vi "FindFaces.vi"() -> ()   [LabVIEW 2018]
panel:
  out "Image to process":picture
  out "Processed image":picture
  out "Error":errorcluster
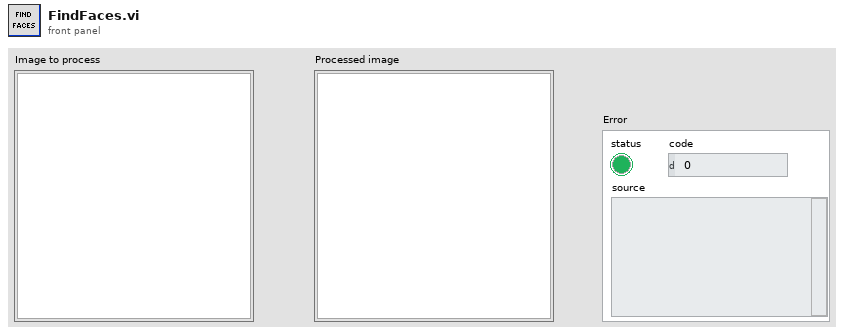
[diagram p1: front panel]
types:
  T1 = typedef "imagedata.ctl" = cluster{"image type":i32, "image depth":i32, "image":u8[], "mask":u8[], "colors":u32[], "Rectangle":cluster{"left":i16, "top":i16, "right":i16, "bottom":i16}}
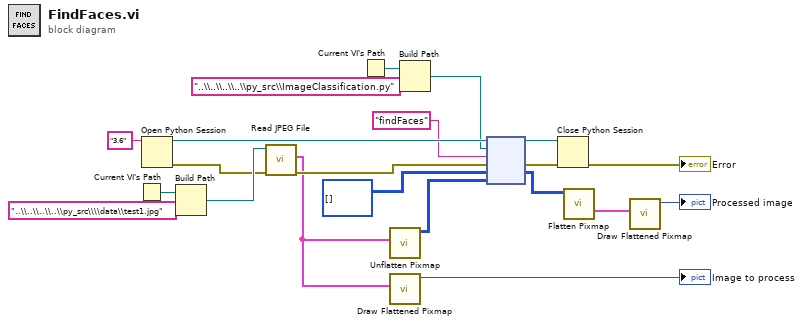
[diagram p0: block diagram]
diagram:
  n1 = Current VI's Path() -> (path=w12:path)
  n2 = Open Python Session(python version="3.6" ("Python version")) -> (session out=w21:refnum<k35>, error out=w7:errorcluster)  [unwired: 2 in]
  n3 = Build Path(base path=w12, name or relative path="..\\..\\..\\..\\py_src\\\\data\\test1.jpg") -> (appended path=w10:path)
  n4 = call <vilib>:"Read JPEG File.vi"("error in (no error)"=w7, "path to JPEG file"=w10) -> ("error out"=w6:errorcluster, "image data"=w4:T1)  [unwired: 7 in, 1 out]
  n5 = Current VI's Path() -> (path=w15:path)
  n6 = call <vilib>:"Unflatten Pixmap.vi"("image data"=w4) -> ("24-bit pixmap"=w1:u32[][])  [unwired: 4 in, 6 out]
  n7 = call <vilib>:"Draw Flattened Pixmap.vi"("image data"=w4) -> ("new picture"=→"Image to process":picture)  [unwired: 8 in]
  n8 = Build Path(base path=w15, name or relative path="..\\..\\..\\..\\py_src\\ImageClassification.py") -> (appended path=w13:path)
  n9 = node(w21, w13, "findFaces" ("function name"), w6, u32[][] [], w1) -> (w20:refnum<k35>, w19:errorcluster, w2:u32[][])  [unwired: 1 in, 2 out]
  n10 = Close Python Session(session in=w20, error in=w19) -> (11:→"Error":errorcluster)
  n11 = call <vilib>:"Flatten Pixmap.vi"("24-bit pixmap"=w2) -> ("image data"=w9:T1)  [unwired: 10 in]
  n12 = call <vilib>:"Draw Flattened Pixmap.vi"("image data"=w9) -> ("new picture"=→"Processed image":picture)  [unwired: 8 in]
